vi "Main.vi"() -> ()   [LabVIEW 2020]
uses:
  <vilib>/Platform/TimedLoop/XDataNode/timing_clust.ctl
  <vilib>/Platform/TimedLoop/XDataNode/nitl_modes.ctl
  <vilib>/Platform/TimedLoop/XDataNode/wakeup.ctl
  <extravilib>/ChannelInstances/Stream-bool/Read With Abort.vi
  <extravilib>/ChannelInstances/Stream-bool/Write With Abort.vi
  <extravilib>/ChannelInstances/Stream-bool/EndpointRead.vi
  <extravilib>/ChannelInstances/Stream-bool/Endpoint.vi
  <extravilib>/ChannelInstances/Stream-bool/Instantiate.vi
  <extravilib>/ChannelInstances/Stream-bool/)Channel.vi
  <resource>/ChannelSupport/_ChannelSupport/WaitIfNeeded.vi
  <extravilib>/ChannelInstances/Event Messenger-str/Instantiate.vi
  <extravilib>/ChannelInstances/Event Messenger-str/))Channel.vi
  <vilib>/platform/TimedLoop/XDataNode/XDataNode.xnode
  <extravilib>/ChannelInstances/Stream-bool.lvlib
  <extravilib>/ChannelInstances/Event Messenger-str.lvlib
  <vilib>/Platform/TimedLoop/XDataNode/XDNodeRunTimeDep.lvlib
panel:
  out "Safety System 1":bool[](array[boolean])
  out "Safety System 2":bool[](array[boolean])
  out "Laser 1":bool
  out "Laser 2":bool
  out "GPS":cluster{"Lat":dbl, "Lon":dbl, "Speed":dbl} {"Lon" format="%#_11g"; "Lat" format="%#_11g"}
  out "Arm System":bool
  in  "Start":bool
  in  "Speed Threshold (km/h)":dbl
  in  "Stop":bool
  out "error out":errorcluster
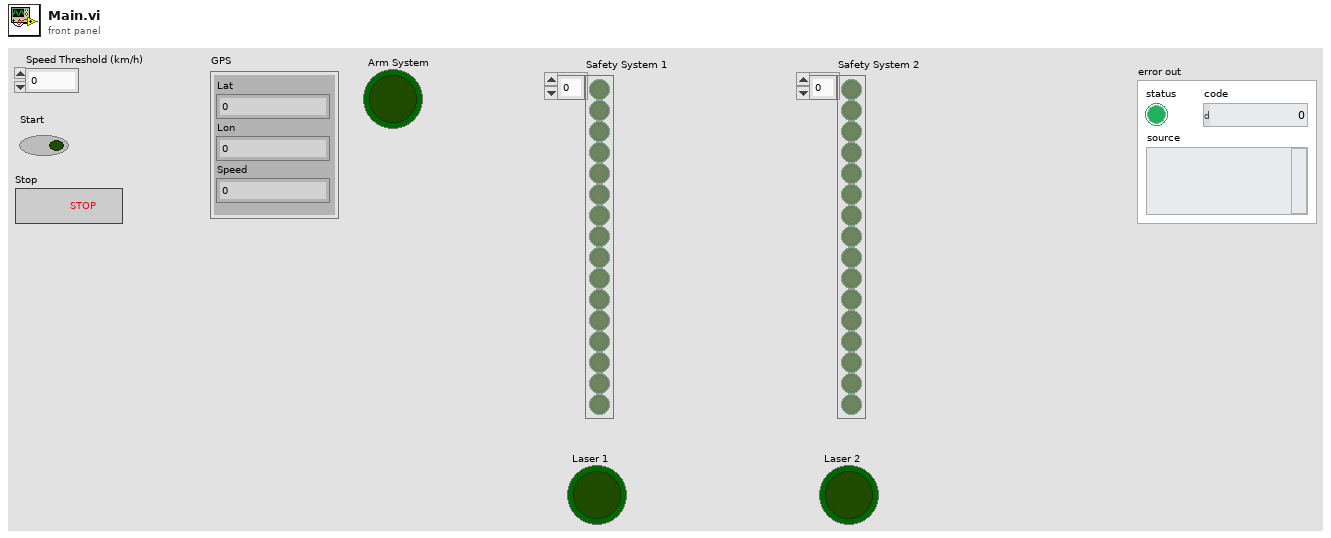
[diagram p1: front panel]
types:
  T1 = enum16{"Initialize", "Wait for Event", "Read TCP Data", "Exit"}
  T2 = typedef "Stream-bool.lvlib/)Channel.ctl" = refnum<queue>
  T3 = enum16{"Standard", "Buffered", "CRLF", "Immediate"}
  T4 = typedef "XDNodeRunTimeDep.lvlib/timing_clust.ctl" = cluster{"Expected End [f-1]":u64, "Actual End [f-1]":u64, "Finished Late? [f-1]":bool, "Expected End [i-1]":u64, "Actual End [i-1]":u64, "Finished Late? [i-1]":bool, "Expected Start [i]":u64, "Actual Start [i]":u64, "Expected Start [f]":u64, "Actual Start [f]":u64, "Source Name":string, "Structure Name":string, "Period":i64, "Deadline":i64, "Offset":i64, "Start":i64, "Priority":i32, "Timeout":i32, "Mode":T5, "Wakeup Reason":T6, "Error":errorcluster, "Source Type":string, "Secondary Source Type":string, "Global End Time":u64, "Global Start Time":u64, "Frame Duration":u64, "Iteration Duration":u64, "Assigned CPU":i32, "I/O Scan Engine Mode":u32}
  T5 = typedef "XDNodeRunTimeDep.lvlib/nitl_modes.ctl" = enum32{"No Change", "Process missed periods, maintain original phase", "Discard missed periods, maintain original phase", "Process missed periods, ignore original phase", "Discard missed periods, ignore original phase"}
  T6 = typedef "XDNodeRunTimeDep.lvlib/wakeup.ctl" = enum32{"Normal", "Aborted", "Asynchronous wakeup", "Timing source error", "Timed loop error", "Timeout"}
  T7 = typedef "Event Messenger-str.lvlib/))Channel.ctl" = refnum<queue>
  T8 = cluster{"event registration refnum":refnum<event-registration>, "event registration refnum":refnum<event-registration>}
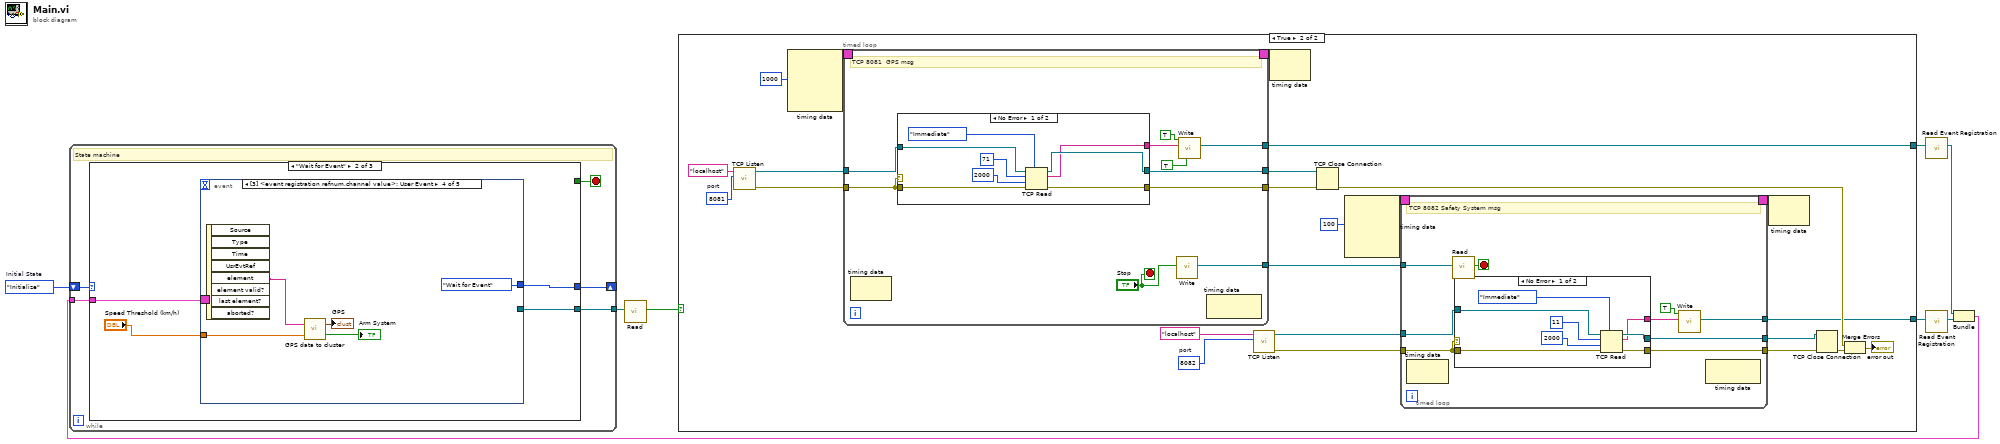
[diagram p0: block diagram]
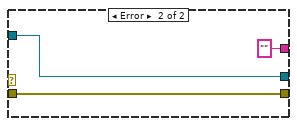
[diagram p3: hidden frame]
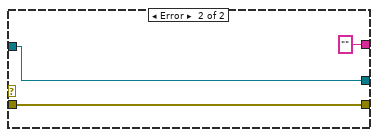
[diagram p4: hidden frame]
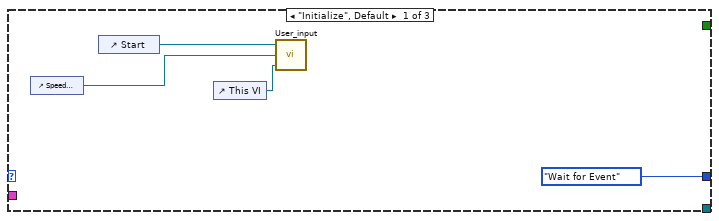
[diagram p5: hidden frame]
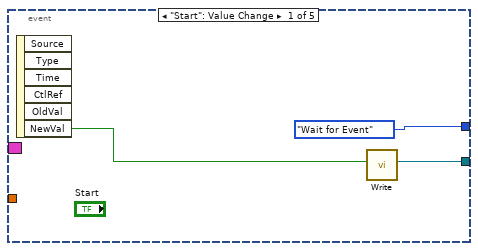
[diagram p6: hidden frame]
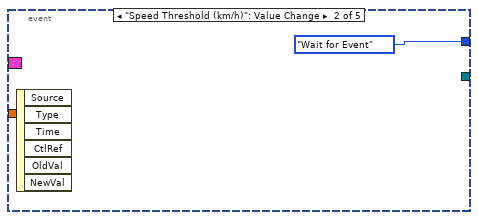
[diagram p7: hidden frame]
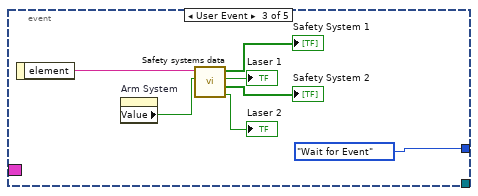
[diagram p8: hidden frame]
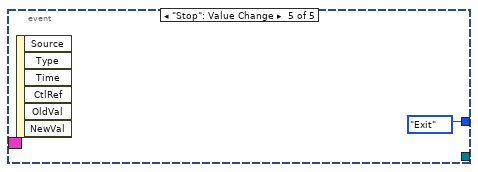
[diagram p9: hidden frame]
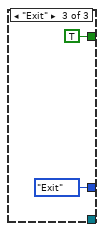
[diagram p10: hidden frame]
diagram:
  w6 = T1."Initialize"  # Initial State
  n1 = while {
    shift-right: [w11] -> _
    shift-left: w6 -> [w13]
    tunnel: w5 -> [w10]
    tunnel: [w9] -> w2
    stop <- w12 stop-if-true
    # "State machine"
    n2 = case shown="\"Wait for Event\"" w13 {
      tunnel: [_ _ TRUE] -> w12
      tunnel: [T1."Wait for Event" ("Initial State") w20 T1."Exit" ("Initial State")] -> w11
      tunnel: w10 -> [_ w19 _]
      tunnel: [_ w21 _] -> w9
      frame "Initialize", Default {
        n3 = control-ref of="Speed Threshold (km/h)"() -> (w16:refnum<vi>)
        n4 = control-ref of="Start"() -> (w15:refnum<vi>)
        n5 = control-ref of="This VI"() -> (w17:refnum<vi>)
        n6 = call "User_input.vi"("Main Vi"=w17, "Speed Threshold (km/h) Ref"=w16, "Start Ref"=w15) -> ()  [unwired: 1 in]
      }
      frame "Wait for Event" {
        n7 = event shown="[3] <event registration refnum.channel value>: User Event" {
          selector: w19 -> [_ _ _ _ _]
          dyn-events: _ -> [_ _ _ _ _]
          timeout: _ -> [_ _ _ _ _]
          tunnel: [w23 _ _ _ _] -> w21
          tunnel: [T1."Wait for Event" ("Initial State") T1."Wait for Event" ("Initial State") T1."Wait for Event" ("Initial State") T1."Wait for Event" ("Initial State") T1."Exit" ("Initial State")] -> w20
          tunnel: "Speed Threshold (km/h)" -> [_ _ _ w35 _]
          event "Start": Value Change {
            n8 = event-data() -> ("NewVal"=w24:bool)  [unwired: 1 in, 5 out]
            n9 = call <extravilib>:"Write.vi"("element"=w24) -> ("channel"=w23:T2)  [unwired: 8 in, 2 out]
          }
          event "Speed Threshold (km/h)": Value Change {
            n10 = event-data() -> ()  [unwired: 1 in, 6 out]
          }
          event User Event {
            n11 = event-data() -> ("element"=w31:string)  [unwired: 1 in]
            n12 = property on="Arm System" class="Bool (strict)"() -> ("Value"=w32:bool)  [unwired: 2 in, 2 out]
            n13 = call "Safety systems data.vi"("Arm System Status"=w32, "safety system raw data"=w31) -> ("Laser 2"=→"Laser 2":bool, "Safety System 2"=→"Safety System 2":bool[], "Laser 1"=→"Laser 1":bool, "Safety System 1"=→"Safety System 1":bool[])  [unwired: 3 in]
          }
          event User Event {
            n14 = event-data() -> ("element"=w34:string)  [unwired: 1 in, 7 out]
            n15 = call "GPS data to cluster.vi"("Speed Threshold (km/h)"=w35, "Gps raw data in"=w34) -> ("Arm System?"=→"Arm System":bool, "GPS Cluster"=→"GPS":cluster{"Lat":dbl, "Lon":dbl, "Speed":dbl})
          }
          event "Stop": Value Change {
            n16 = event-data() -> ()  [unwired: 1 in, 6 out]
          }
        }
      }
      frame "Exit" {
      }
    }
  }
  n17 = call <extravilib>:"Read.vi"("channel"=w2) -> ("element"=w1:bool)  [unwired: 6 in, 4 out]
  n18 = case shown="True" w1 {
    tunnel: [_ w42] -> w4
    tunnel: [_ w41] -> w3
    frame False {
    }
    frame True {
      w54 = u16 8082  # port
      w60 = u16 8081  # port
      n19 = call <vilib>:"TCP Listen.vi"("port"=w60, "service name"="localhost") -> ("error out"=w58:errorcluster, "connection ID"=w51:refnum<k5>)  [unwired: 5 in, 3 out]
      n20 = node-c288(i64 1000 ("Period")) -> (w64:T4)  [unwired: 3 in]
      n21 = timed-loop {
        tunnel: w58 -> [w97]
        tunnel: w51 -> [w100]
        tunnel: [w99] -> w50
        tunnel: [w98] -> w49
        timing: w64 -> [_]
        timing-out: [_] -> w63
        tunnel: [w96] -> w43
        tunnel: [w94] -> w42
        stop <- "Stop" stop-if-true
        # "TCP 8081  GPS msg"
        n22 = node-c288() -> ()  [unwired: 1 in, 1 out]
        n23 = case shown="No Error" w97 {
          tunnel: w97 -> [w105 w111]
          tunnel: w100 -> [w104 w110]
          tunnel: [w103 w111] -> w99
          tunnel: [w102 w110] -> w98
          tunnel: [w101 "" ("data out")] -> w95
          frame No Error {
            n24 = TCP Read(connection ID=w104, bytes to read=71, error in (no error)=w105, 7:T3."Immediate" ("mode (standard)"), 9:2000 ("timeout ms (25000)")) -> (connection ID out=w102:refnum<k5>, data out=w101:string, error out=w103:errorcluster)
          }
          frame Error {
          }
        }
        n25 = call <extravilib>:"Write.vi"("element"="Stop") -> ("channel"=w96:T2)  [unwired: 8 in, 2 out]
        n26 = call <extravilib>:"Write.vi"("high priority? (F)"=TRUE, "element"=w95, "element valid? (T)"=TRUE) -> ("channel"=w94:T7)  [unwired: 7 in, 1 out]
        n27 = node-c288() -> ()  [unwired: 1 in, 1 out]
      }
      n28 = call <vilib>:"TCP Listen.vi"("port"=w54, "service name"="localhost") -> ("error out"=w56:errorcluster, "connection ID"=w57:refnum<k5>)  [unwired: 5 in, 3 out]
      n29 = node-c288(w63) -> ()  [unwired: 1 out]
      n30 = TCP Close Connection(connection ID=w49, error in (no error)=w50) -> (error out=w45:errorcluster)  [unwired: 1 in, 1 out]
      n31 = node-c288(i64 100 ("Period")) -> (w62:T4)  [unwired: 3 in]
      n32 = timed-loop {
        tunnel: w56 -> [w70]
        tunnel: w57 -> [w73]
        tunnel: [w72] -> w48
        tunnel: [w71] -> w47
        timing: w62 -> [_]
        timing-out: [_] -> w61
        tunnel: w43 -> [w68]
        tunnel: [w66] -> w41
        stop <- w69 stop-if-true
        # "TCP 8082 Safety System msg"
        n33 = node-c288() -> ()  [unwired: 1 in, 1 out]
        n34 = call <extravilib>:"Read.vi"("channel"=w68) -> ("element"=w69:bool)  [unwired: 6 in, 4 out]
        n35 = case shown="No Error" w70 {
          tunnel: w70 -> [w78 w84]
          tunnel: w73 -> [w77 w83]
          tunnel: [w76 w84] -> w72
          tunnel: [w75 w83] -> w71
          tunnel: [w74 "" ("data out")] -> w67
          frame No Error {
            n36 = TCP Read(connection ID=w77, bytes to read=11, error in (no error)=w78, 7:T3."Immediate" ("mode (standard)"), 9:2000 ("timeout ms (25000)")) -> (connection ID out=w75:refnum<k5>, data out=w74:string, error out=w76:errorcluster)
          }
          frame Error {
          }
        }
        n37 = call <extravilib>:"Write.vi"("element"=w67, "element valid? (T)"=TRUE) -> ("channel"=w66:T7)  [unwired: 8 in, 1 out]
        n38 = node-c288() -> ()  [unwired: 1 in, 1 out]
      }
      n39 = node-c288(w61) -> ()  [unwired: 1 out]
      n40 = TCP Close Connection(connection ID=w47, error in (no error)=w48) -> (error out=w44:errorcluster)  [unwired: 1 in, 1 out]
      n41 = Merge Errors(w45, w44) -> (→"error out":errorcluster)
    }
  }
  n42 = call <extravilib>:"Read Event Registration.vi"("channel"=w4) -> ("event registration refnum"=w7:refnum<event-registration>)  [unwired: 10 in]
  n43 = call <extravilib>:"Read Event Registration.vi"("channel"=w3) -> ("event registration refnum"=w8:refnum<event-registration>)  [unwired: 10 in]
  n44 = Bundle("event registration refnum"=w7, "event registration refnum"=w8) -> (w5:T8)  [unwired: 1 in]
